vi "speak.vi"(8 "error in (no error)":errorcluster, 11 "Animal in":refnum<class "IAnimal.lvclass">) -> (0 "error out":errorcluster, 3 "Animal out":refnum<class "IAnimal.lvclass">)   [LabVIEW 2024, in "IAnimal.lvclass"]
uses:
  IAnimal.lvclass
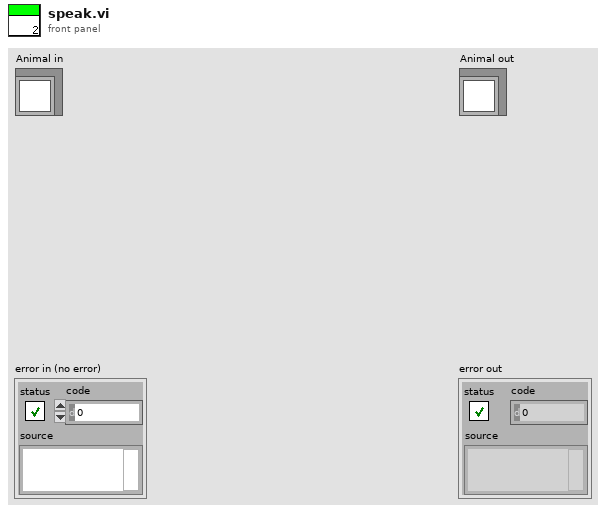
[diagram p1: front panel]
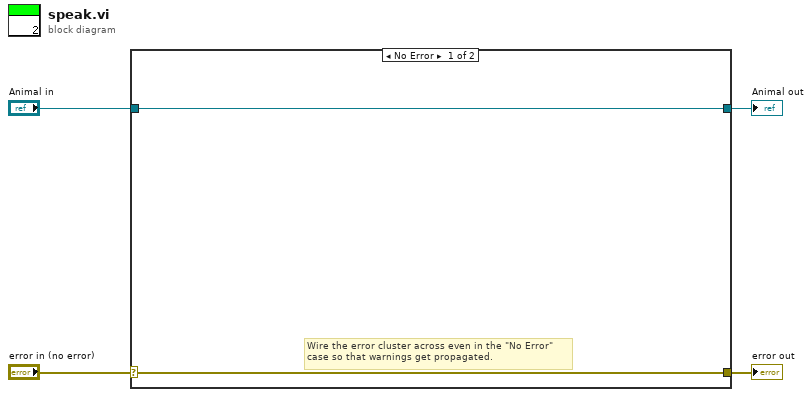
[diagram p0: block diagram]
diagram:
  n1 = case shown="No Error" "error in (no error)" {
    selector: "error in (no error)" -> [w5 w8]
    tunnel: [w5 w8] -> w3
    tunnel: [w6 w7] -> w1
    tunnel: "Animal in" -> [w6 w7]
    frame No Error {
      # "Wire the error cluster across even in the \"No Error\"\ncase so that warnings get propagated."
    }
    frame Error {
    }
  }
  "error out" <- w3
  "Animal out" <- w1
